vi "Check Should Update View.vi"(8 "error in (no error)":errorcluster, 11 "ConsoleView in":refnum<class "ConsoleView.lvclass">) -> (0 "error out":errorcluster, 2 "Log?":bool, 3 "ConsoleView out":refnum<class "ConsoleView.lvclass">)   [LabVIEW 2017, in "ConsoleView.lvlib" / "ConsoleView.lvclass"]
uses:
  ConsoleView.lvclass
  ConsoleView.lvclass/ConsoleView.ctl
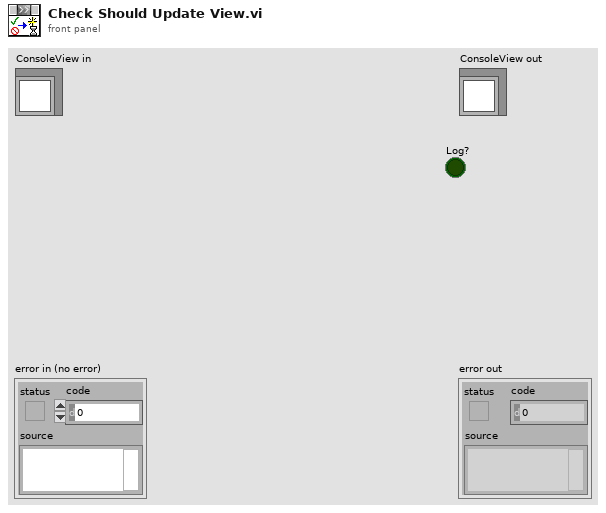
[diagram p1: front panel]
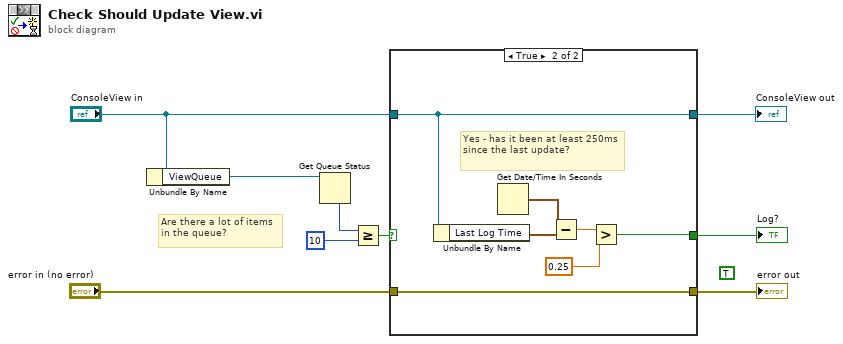
[diagram p0: block diagram]
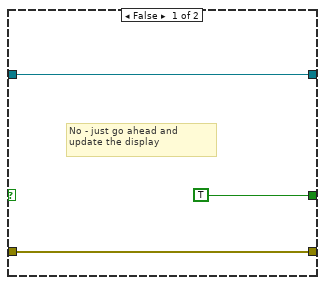
[diagram p2: hidden frame]
diagram:
  (unwired) TRUE ("Log?")
  # "Are there a lot of items in the queue?"
  n1 = Unbundle By Name("ConsoleView in") -> ("ViewQueue"=w9:refnum<queue>)
  n2 = Get Queue Status(queue=w9) -> (# elements in queue=w8:i32)  [unwired: 2 in, 7 out]
  n3 = Greater Or Equal?(x=w8, y=10) -> (x >= y?=w6:bool)
  n4 = case shown="True" w6 {
    tunnel: "ConsoleView in" -> [w12 w18]
    tunnel: [w12 w18] -> w2
    tunnel: "error in (no error)" -> [w11 w19]
    tunnel: [w11 w19] -> w3
    tunnel: [TRUE w13] -> w1
    frame False {
      # "No - just go ahead and update the display"
    }
    frame True {
      # "Yes - has it been at least 250ms since the last update?"
      n5 = Unbundle By Name(w18) -> ("Last Log Time"=w17:timestamp)
      n6 = Get Date/Time In Seconds() -> (seconds since 1Jan1904=w16:timestamp)
      n7 = Subtract(x=w16, y=w17) -> (x-y=w15:dbl)
      n8 = Greater?(x=w15, y=0.25) -> (0:w13:bool)
    }
  }
  "error out" <- w3
  "ConsoleView out" <- w2
  "Log?" <- w1
